vi "ArmPathPlannerStateMachine.vi"() -> ()   [LabVIEW 2017]
uses:
  TypeDefs/ArmState_TypeDef.ctl
  General/PathPlanning/TypeDefs/Point2D.ctl
  TypeDefs/ArmCoordinate.ctl
panel:
  in  "MaxArmExtension":dbl
  in  "MinArmExtension":dbl
  in  "EndPoint":T1
  out "OutputArmPoint":T2
  in  "StartPoint":T1
  in  "Extend Finish":bool
  in  "Pivot Finished":bool
  in  "Retract Finished":bool
  in  "Start":bool
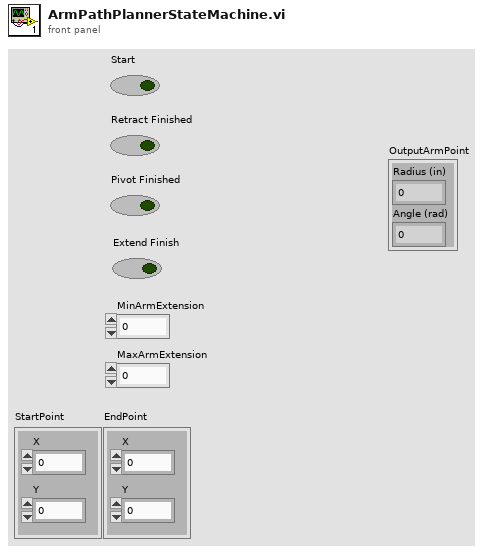
[diagram p1: front panel]
types:
  T1 = typedef "Point2D.ctl" = cluster{"X":dbl, "Y":dbl}
  T2 = typedef "ArmCoordinate.ctl" = cluster{"Radius (in)":dbl, "Angle (rad)":dbl}
  T3 = typedef "ArmState_TypeDef.ctl" = enum16{"Retract ", "Pivot ", "Extend ", "Idle "}
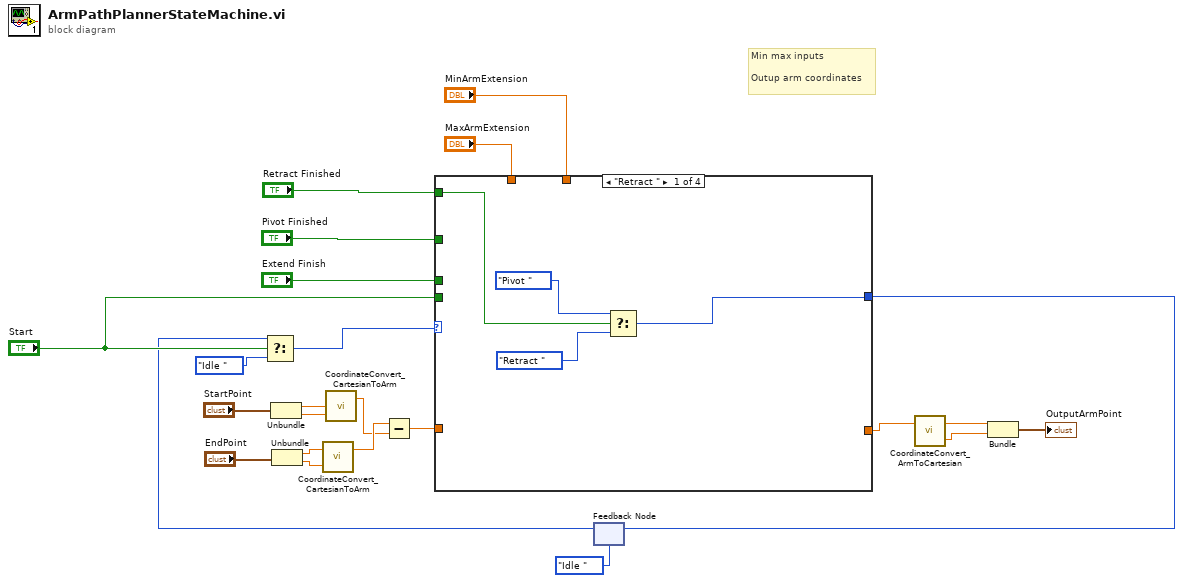
[diagram p0: block diagram]
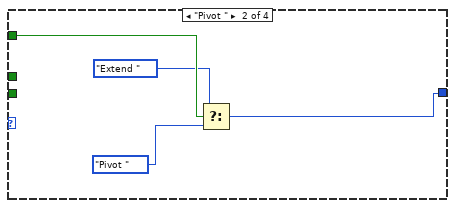
[diagram p2: hidden frame]
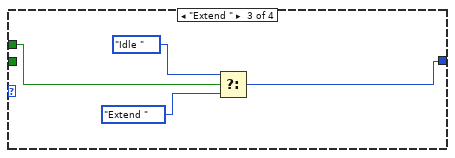
[diagram p3: hidden frame]
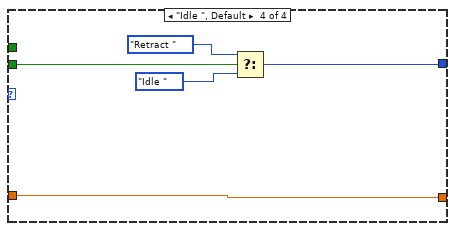
[diagram p4: hidden frame]
diagram:
  # "Min max inputs \n\nOutup arm coordinates"
  n1 = Unbundle("StartPoint") -> ("X"=w14:dbl, "Y"=w13:dbl)
  n2 = Unbundle("EndPoint") -> ("X"=w12:dbl, "Y"=w11:dbl)
  n3 = call "CoordinateConvert_CartesianToArm.vi"("Y (in)"=w11, "X (in)"=w12) -> ("Angle (rad)"=w9:dbl)  [unwired: 1 out]
  n4 = call "CoordinateConvert_CartesianToArm.vi"("Y (in)"=w13, "X (in)"=w14) -> ("Angle (rad)"=w8:dbl)  [unwired: 1 out]
  n5 = Subtract(x=w9, y=w8) -> (x-y=w7:dbl)
  n6 = feedback #1(ArmState_TypeDef."Idle " ("Enum")) -> (w20:T3)
  n7 = Select(t=w20, s="Start", f=ArmState_TypeDef."Idle " ("Enum")) -> (s? t:f=w23:T3)
  n8 = case shown="\"Retract \"" w23 {
    tunnel: "Start" -> [_ _ _ w41]
    tunnel: [w25 w29 w35 w38] -> w21
    tunnel: "Retract Finished" -> [w28 _ _ _]
    tunnel: "Pivot Finished" -> [_ w32 _ _]
    tunnel: "Extend Finish" -> [_ _ w36 _]
    tunnel: w7 -> [_ _ _ w37]
    tunnel: [_ _ _ w37] -> w3
    tunnel: "MinArmExtension" -> [_ _ _ _]
    tunnel: "MaxArmExtension" -> [_ _ _ _]
    frame "Retract " {
      n9 = Select(t=ArmState_TypeDef."Pivot " ("Enum"), s=w28, f=ArmState_TypeDef."Retract " ("Enum")) -> (s? t:f=w25:T3)
    }
    frame "Pivot " {
      n10 = Select(t=ArmState_TypeDef."Extend " ("Enum"), s=w32, f=ArmState_TypeDef."Pivot " ("Enum")) -> (s? t:f=w29:T3)
    }
    frame "Extend " {
      n11 = Select(t=ArmState_TypeDef."Idle " ("Enum"), s=w36, f=ArmState_TypeDef."Extend " ("Enum")) -> (s? t:f=w35:T3)
    }
    frame "Idle ", Default {
      n12 = Select(t=ArmState_TypeDef."Retract " ("Enum"), s=w41, f=ArmState_TypeDef."Idle " ("Enum")) -> (s? t:f=w38:T3)
    }
  }
  n13 = feedback-in #1(w21) -> ()
  n14 = call "CoordinateConvert_ArmToCartesian.vi"("Angle (rad)"=w3) -> ("Y (in)"=w5:dbl, "X (in)"=w6:dbl)  [unwired: 1 in]
  n15 = Bundle("X (in)"=w6, "Y (in)"=w5) -> (→"OutputArmPoint":cluster{"X (in)":dbl, "Y (in)":dbl})  [unwired: 1 in]
